vi "Auton Data.vi"(8 "power":dbl[](array[numeric]), 9 "time/distance":dbl[](array[numeric]), 10 "Heading":dbl[](array[numeric]), 11 "primitive ID":i16[](array[numeric])) -> ()   [LabVIEW 2012]
uses:
  <vilib>/Rock Robotics/WPI/DriverStation/DriverStationLCD/WPI_DriverStationLCDLCDLine.ctl
  Begin/Global Variables.vi
panel:
  out "Heading":dbl
  out "Distance/Time":dbl
  out "Power":dbl
  out "ArrayIndex":u16
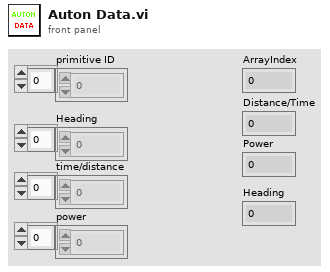
[diagram p1: front panel]
types:
  T1 = typedef "WPI_DriverStationLCDLCDLine.ctl" = enum16{"Main - Line 1", "User - Line 2", "User - Line 3", "User - Line 4", "User - Line 5", "User - Line 6"}
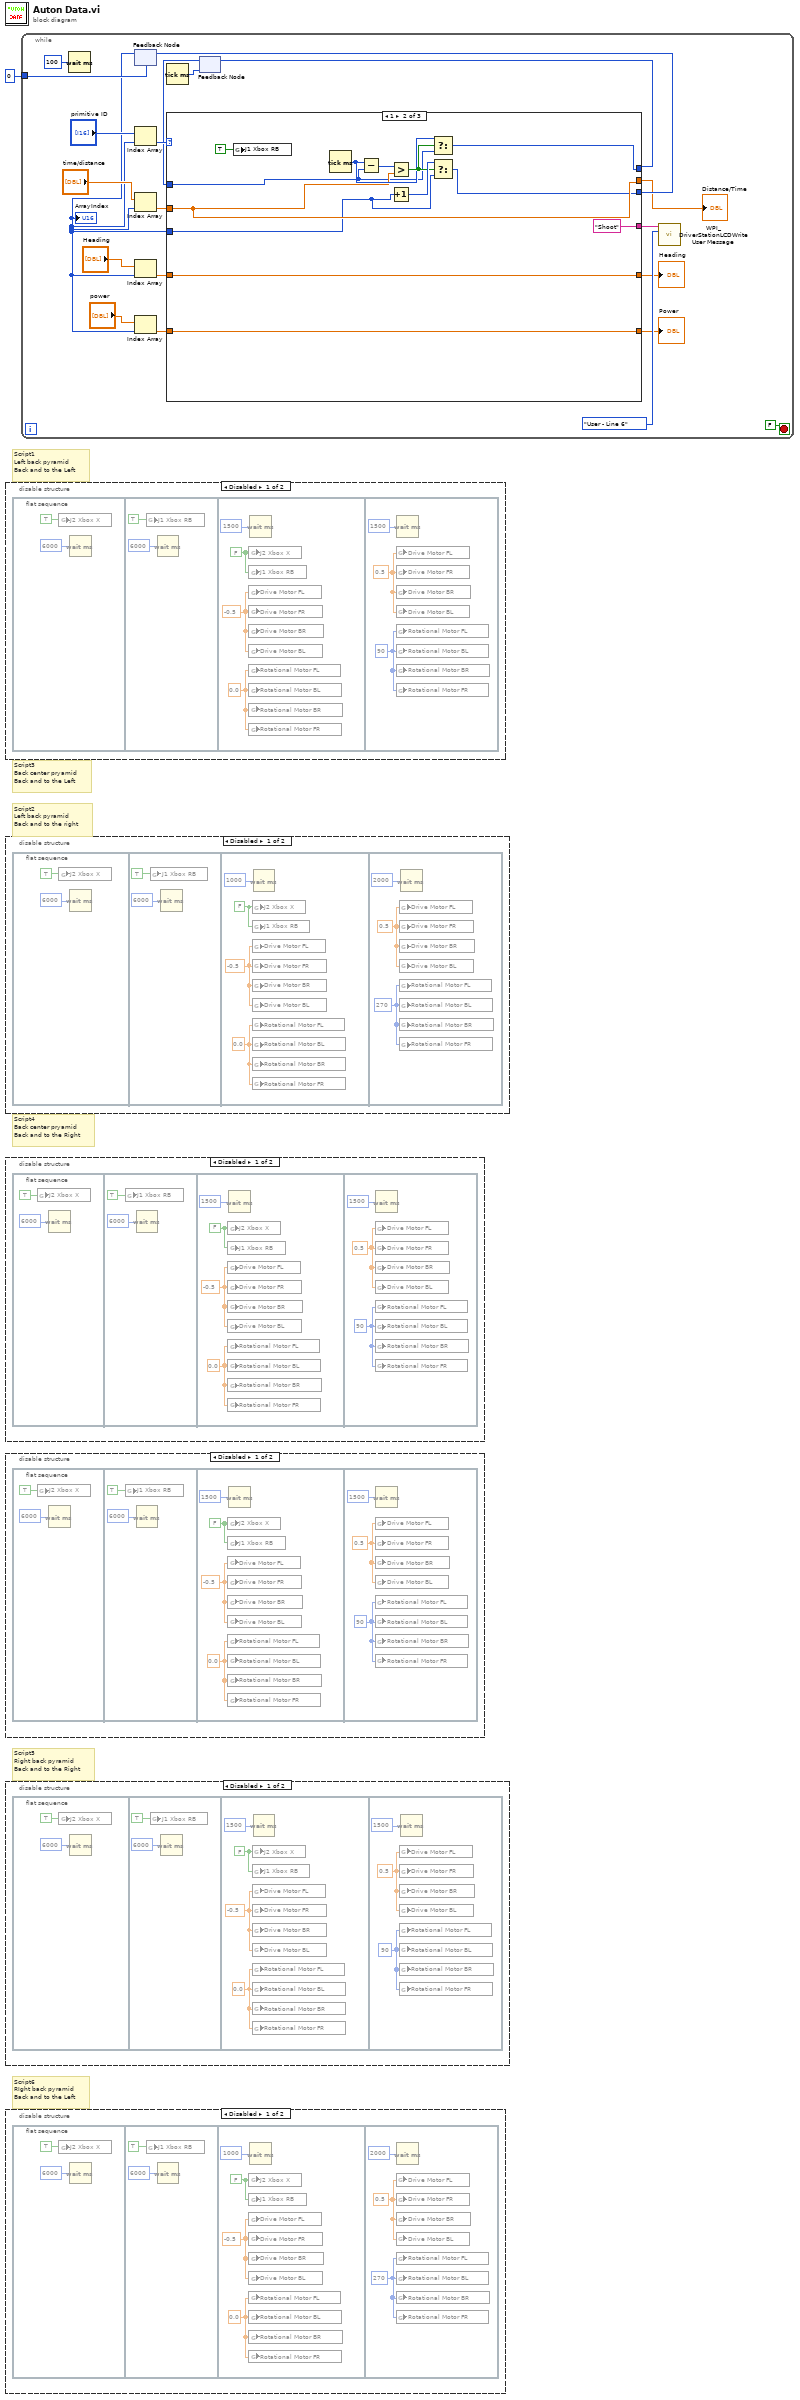
[diagram p0: block diagram]
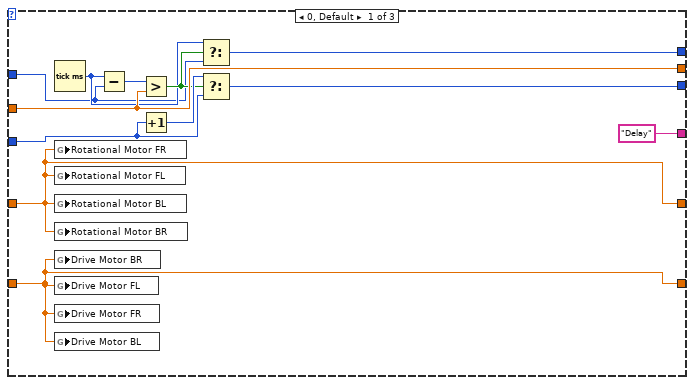
[diagram p2: hidden frame]
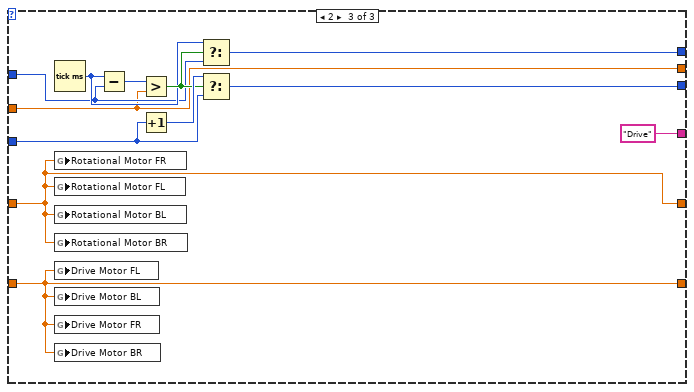
[diagram p3: hidden frame]
diagram:
  # "Script6\nRIght back pyramid\nBack and to the Left"
  # "Script5\nRight back pyramid\nBack and to the Right"
  # "Script4\nBack center pryamid\nBack and to the Right"
  # "Script3\nBack center pryamid\nBack and to the Left"
  # "Script2\nLeft back pyramid\nBack and to the right"
  # "Script1\nLeft back pyramid\nBack and to the Left"
  n1 = disable-structure shown="Disabled" {
    frame Disabled {
      n2 = flat-sequence {
        frame #0 {
          n3 = global write "Global Variables.vi" "J2 Xbox X"(TRUE) -> ()
          n4 = Wait (ms)(milliseconds to wait=u32 6000) -> ()  [unwired: 1 out]
        }
        frame #1 {
          n5 = global write "Global Variables.vi" "J1 Xbox RB"(TRUE ("Shoot trigger")) -> ()
          n6 = Wait (ms)(milliseconds to wait=u32 6000) -> ()  [unwired: 1 out]
        }
        frame #2 {
          w8 = -0.5
          w9 = 0.0
          w6 = FALSE ("Shoot trigger")
          n7 = global write "Global Variables.vi" "J2 Xbox X"(w6) -> ()
          n8 = global write "Global Variables.vi" "J1 Xbox RB"(w6) -> ()
          n9 = global write "Global Variables.vi" "Drive Motor FL"(w8) -> ()
          n10 = global write "Global Variables.vi" "Drive Motor FR"(w8) -> ()
          n11 = global write "Global Variables.vi" "Drive Motor BR"(w8) -> ()
          n12 = global write "Global Variables.vi" "Drive Motor BL"(w8) -> ()
          n13 = global write "Global Variables.vi" "Rotational Motor FL"(w9) -> ()
          n14 = global write "Global Variables.vi" "Rotational Motor BL"(w9) -> ()
          n15 = global write "Global Variables.vi" "Rotational Motor BR"(w9) -> ()
          n16 = global write "Global Variables.vi" "Rotational Motor FR"(w9) -> ()
          n17 = Wait (ms)(milliseconds to wait=u32 1500) -> ()  [unwired: 1 out]
        }
        frame #3 {
          w11 = 0.5
          w10 = 90
          n18 = global write "Global Variables.vi" "Drive Motor FL"(w11) -> ()
          n19 = global write "Global Variables.vi" "Drive Motor FR"(w11) -> ()
          n20 = global write "Global Variables.vi" "Drive Motor BR"(w11) -> ()
          n21 = global write "Global Variables.vi" "Drive Motor BL"(w11) -> ()
          n22 = global write "Global Variables.vi" "Rotational Motor FL"(w10) -> ()
          n23 = global write "Global Variables.vi" "Rotational Motor BL"(w10) -> ()
          n24 = global write "Global Variables.vi" "Rotational Motor BR"(w10) -> ()
          n25 = global write "Global Variables.vi" "Rotational Motor FR"(w10) -> ()
          n26 = Wait (ms)(milliseconds to wait=u32 1500) -> ()  [unwired: 1 out]
        }
      }
    }
    frame Enabled {
    }
  }
  n27 = disable-structure shown="Disabled" {
    frame Disabled {
      n28 = flat-sequence {
        frame #0 {
          n29 = global write "Global Variables.vi" "J2 Xbox X"(TRUE) -> ()
          n30 = Wait (ms)(milliseconds to wait=u32 6000) -> ()  [unwired: 1 out]
        }
        frame #1 {
          n31 = global write "Global Variables.vi" "J1 Xbox RB"(TRUE ("Shoot trigger")) -> ()
          n32 = Wait (ms)(milliseconds to wait=u32 6000) -> ()  [unwired: 1 out]
        }
        frame #2 {
          w19 = -0.5
          w20 = 0.0
          w17 = FALSE ("Shoot trigger")
          n33 = global write "Global Variables.vi" "J2 Xbox X"(w17) -> ()
          n34 = global write "Global Variables.vi" "J1 Xbox RB"(w17) -> ()
          n35 = global write "Global Variables.vi" "Drive Motor FL"(w19) -> ()
          n36 = global write "Global Variables.vi" "Drive Motor FR"(w19) -> ()
          n37 = global write "Global Variables.vi" "Drive Motor BR"(w19) -> ()
          n38 = global write "Global Variables.vi" "Drive Motor BL"(w19) -> ()
          n39 = global write "Global Variables.vi" "Rotational Motor FL"(w20) -> ()
          n40 = global write "Global Variables.vi" "Rotational Motor BL"(w20) -> ()
          n41 = global write "Global Variables.vi" "Rotational Motor BR"(w20) -> ()
          n42 = global write "Global Variables.vi" "Rotational Motor FR"(w20) -> ()
          n43 = Wait (ms)(milliseconds to wait=u32 1000) -> ()  [unwired: 1 out]
        }
        frame #3 {
          w22 = 0.5
          w21 = 270
          n44 = global write "Global Variables.vi" "Drive Motor FL"(w22) -> ()
          n45 = global write "Global Variables.vi" "Drive Motor FR"(w22) -> ()
          n46 = global write "Global Variables.vi" "Drive Motor BR"(w22) -> ()
          n47 = global write "Global Variables.vi" "Drive Motor BL"(w22) -> ()
          n48 = global write "Global Variables.vi" "Rotational Motor FL"(w21) -> ()
          n49 = global write "Global Variables.vi" "Rotational Motor BL"(w21) -> ()
          n50 = global write "Global Variables.vi" "Rotational Motor BR"(w21) -> ()
          n51 = global write "Global Variables.vi" "Rotational Motor FR"(w21) -> ()
          n52 = Wait (ms)(milliseconds to wait=u32 2000) -> ()  [unwired: 1 out]
        }
      }
    }
    frame Enabled {
    }
  }
  n53 = disable-structure shown="Disabled" {
    frame Disabled {
      n54 = flat-sequence {
        frame #0 {
          n55 = global write "Global Variables.vi" "J2 Xbox X"(TRUE) -> ()
          n56 = Wait (ms)(milliseconds to wait=u32 6000) -> ()  [unwired: 1 out]
        }
        frame #1 {
          n57 = global write "Global Variables.vi" "J1 Xbox RB"(TRUE ("Shoot trigger")) -> ()
          n58 = Wait (ms)(milliseconds to wait=u32 6000) -> ()  [unwired: 1 out]
        }
        frame #2 {
          w30 = -0.5
          w31 = 0.0
          w28 = FALSE ("Shoot trigger")
          n59 = global write "Global Variables.vi" "J2 Xbox X"(w28) -> ()
          n60 = global write "Global Variables.vi" "J1 Xbox RB"(w28) -> ()
          n61 = global write "Global Variables.vi" "Drive Motor FL"(w30) -> ()
          n62 = global write "Global Variables.vi" "Drive Motor FR"(w30) -> ()
          n63 = global write "Global Variables.vi" "Drive Motor BR"(w30) -> ()
          n64 = global write "Global Variables.vi" "Drive Motor BL"(w30) -> ()
          n65 = global write "Global Variables.vi" "Rotational Motor FL"(w31) -> ()
          n66 = global write "Global Variables.vi" "Rotational Motor BL"(w31) -> ()
          n67 = global write "Global Variables.vi" "Rotational Motor BR"(w31) -> ()
          n68 = global write "Global Variables.vi" "Rotational Motor FR"(w31) -> ()
          n69 = Wait (ms)(milliseconds to wait=u32 1500) -> ()  [unwired: 1 out]
        }
        frame #3 {
          w33 = 0.5
          w32 = 90
          n70 = global write "Global Variables.vi" "Drive Motor FL"(w33) -> ()
          n71 = global write "Global Variables.vi" "Drive Motor FR"(w33) -> ()
          n72 = global write "Global Variables.vi" "Drive Motor BR"(w33) -> ()
          n73 = global write "Global Variables.vi" "Drive Motor BL"(w33) -> ()
          n74 = global write "Global Variables.vi" "Rotational Motor FL"(w32) -> ()
          n75 = global write "Global Variables.vi" "Rotational Motor BL"(w32) -> ()
          n76 = global write "Global Variables.vi" "Rotational Motor BR"(w32) -> ()
          n77 = global write "Global Variables.vi" "Rotational Motor FR"(w32) -> ()
          n78 = Wait (ms)(milliseconds to wait=u32 1500) -> ()  [unwired: 1 out]
        }
      }
    }
    frame Enabled {
    }
  }
  n79 = disable-structure shown="Disabled" {
    frame Disabled {
      n80 = flat-sequence {
        frame #0 {
          n81 = global write "Global Variables.vi" "J2 Xbox X"(TRUE) -> ()
          n82 = Wait (ms)(milliseconds to wait=u32 6000) -> ()  [unwired: 1 out]
        }
        frame #1 {
          n83 = global write "Global Variables.vi" "J1 Xbox RB"(TRUE ("Shoot trigger")) -> ()
          n84 = Wait (ms)(milliseconds to wait=u32 6000) -> ()  [unwired: 1 out]
        }
        frame #2 {
          w41 = -0.5
          w42 = 0.0
          w39 = FALSE ("Shoot trigger")
          n85 = global write "Global Variables.vi" "J2 Xbox X"(w39) -> ()
          n86 = global write "Global Variables.vi" "J1 Xbox RB"(w39) -> ()
          n87 = global write "Global Variables.vi" "Drive Motor FL"(w41) -> ()
          n88 = global write "Global Variables.vi" "Drive Motor FR"(w41) -> ()
          n89 = global write "Global Variables.vi" "Drive Motor BR"(w41) -> ()
          n90 = global write "Global Variables.vi" "Drive Motor BL"(w41) -> ()
          n91 = global write "Global Variables.vi" "Rotational Motor FL"(w42) -> ()
          n92 = global write "Global Variables.vi" "Rotational Motor BL"(w42) -> ()
          n93 = global write "Global Variables.vi" "Rotational Motor BR"(w42) -> ()
          n94 = global write "Global Variables.vi" "Rotational Motor FR"(w42) -> ()
          n95 = Wait (ms)(milliseconds to wait=u32 1500) -> ()  [unwired: 1 out]
        }
        frame #3 {
          w44 = 0.5
          w43 = 90
          n96 = global write "Global Variables.vi" "Drive Motor FL"(w44) -> ()
          n97 = global write "Global Variables.vi" "Drive Motor FR"(w44) -> ()
          n98 = global write "Global Variables.vi" "Drive Motor BR"(w44) -> ()
          n99 = global write "Global Variables.vi" "Drive Motor BL"(w44) -> ()
          n100 = global write "Global Variables.vi" "Rotational Motor FL"(w43) -> ()
          n101 = global write "Global Variables.vi" "Rotational Motor BL"(w43) -> ()
          n102 = global write "Global Variables.vi" "Rotational Motor BR"(w43) -> ()
          n103 = global write "Global Variables.vi" "Rotational Motor FR"(w43) -> ()
          n104 = Wait (ms)(milliseconds to wait=u32 1500) -> ()  [unwired: 1 out]
        }
      }
    }
    frame Enabled {
    }
  }
  n105 = disable-structure shown="Disabled" {
    frame Disabled {
      n106 = flat-sequence {
        frame #0 {
          n107 = global write "Global Variables.vi" "J2 Xbox X"(TRUE) -> ()
          n108 = Wait (ms)(milliseconds to wait=u32 6000) -> ()  [unwired: 1 out]
        }
        frame #1 {
          n109 = global write "Global Variables.vi" "J1 Xbox RB"(TRUE ("Shoot trigger")) -> ()
          n110 = Wait (ms)(milliseconds to wait=u32 6000) -> ()  [unwired: 1 out]
        }
        frame #2 {
          w52 = -0.5
          w53 = 0.0
          w50 = FALSE ("Shoot trigger")
          n111 = global write "Global Variables.vi" "J2 Xbox X"(w50) -> ()
          n112 = global write "Global Variables.vi" "J1 Xbox RB"(w50) -> ()
          n113 = global write "Global Variables.vi" "Drive Motor FL"(w52) -> ()
          n114 = global write "Global Variables.vi" "Drive Motor FR"(w52) -> ()
          n115 = global write "Global Variables.vi" "Drive Motor BR"(w52) -> ()
          n116 = global write "Global Variables.vi" "Drive Motor BL"(w52) -> ()
          n117 = global write "Global Variables.vi" "Rotational Motor FL"(w53) -> ()
          n118 = global write "Global Variables.vi" "Rotational Motor BL"(w53) -> ()
          n119 = global write "Global Variables.vi" "Rotational Motor BR"(w53) -> ()
          n120 = global write "Global Variables.vi" "Rotational Motor FR"(w53) -> ()
          n121 = Wait (ms)(milliseconds to wait=u32 1500) -> ()  [unwired: 1 out]
        }
        frame #3 {
          w55 = 0.5
          w54 = 90
          n122 = global write "Global Variables.vi" "Drive Motor FL"(w55) -> ()
          n123 = global write "Global Variables.vi" "Drive Motor FR"(w55) -> ()
          n124 = global write "Global Variables.vi" "Drive Motor BR"(w55) -> ()
          n125 = global write "Global Variables.vi" "Drive Motor BL"(w55) -> ()
          n126 = global write "Global Variables.vi" "Rotational Motor FL"(w54) -> ()
          n127 = global write "Global Variables.vi" "Rotational Motor BL"(w54) -> ()
          n128 = global write "Global Variables.vi" "Rotational Motor BR"(w54) -> ()
          n129 = global write "Global Variables.vi" "Rotational Motor FR"(w54) -> ()
          n130 = Wait (ms)(milliseconds to wait=u32 1500) -> ()  [unwired: 1 out]
        }
      }
    }
    frame Enabled {
    }
  }
  n131 = disable-structure shown="Disabled" {
    frame Disabled {
      n132 = flat-sequence {
        frame #0 {
          n133 = global write "Global Variables.vi" "J2 Xbox X"(TRUE) -> ()
          n134 = Wait (ms)(milliseconds to wait=u32 6000) -> ()  [unwired: 1 out]
        }
        frame #1 {
          n135 = global write "Global Variables.vi" "J1 Xbox RB"(TRUE ("Shoot trigger")) -> ()
          n136 = Wait (ms)(milliseconds to wait=u32 6000) -> ()  [unwired: 1 out]
        }
        frame #2 {
          w63 = -0.5
          w64 = 0.0
          w61 = FALSE ("Shoot trigger")
          n137 = global write "Global Variables.vi" "J2 Xbox X"(w61) -> ()
          n138 = global write "Global Variables.vi" "J1 Xbox RB"(w61) -> ()
          n139 = global write "Global Variables.vi" "Drive Motor FL"(w63) -> ()
          n140 = global write "Global Variables.vi" "Drive Motor FR"(w63) -> ()
          n141 = global write "Global Variables.vi" "Drive Motor BR"(w63) -> ()
          n142 = global write "Global Variables.vi" "Drive Motor BL"(w63) -> ()
          n143 = global write "Global Variables.vi" "Rotational Motor FL"(w64) -> ()
          n144 = global write "Global Variables.vi" "Rotational Motor BL"(w64) -> ()
          n145 = global write "Global Variables.vi" "Rotational Motor BR"(w64) -> ()
          n146 = global write "Global Variables.vi" "Rotational Motor FR"(w64) -> ()
          n147 = Wait (ms)(milliseconds to wait=u32 1000) -> ()  [unwired: 1 out]
        }
        frame #3 {
          w66 = 0.5
          w65 = 270
          n148 = global write "Global Variables.vi" "Drive Motor FL"(w66) -> ()
          n149 = global write "Global Variables.vi" "Drive Motor FR"(w66) -> ()
          n150 = global write "Global Variables.vi" "Drive Motor BR"(w66) -> ()
          n151 = global write "Global Variables.vi" "Drive Motor BL"(w66) -> ()
          n152 = global write "Global Variables.vi" "Rotational Motor FL"(w65) -> ()
          n153 = global write "Global Variables.vi" "Rotational Motor BL"(w65) -> ()
          n154 = global write "Global Variables.vi" "Rotational Motor BR"(w65) -> ()
          n155 = global write "Global Variables.vi" "Rotational Motor FR"(w65) -> ()
          n156 = Wait (ms)(milliseconds to wait=u32 2000) -> ()  [unwired: 1 out]
        }
      }
    }
    frame Enabled {
    }
  }
  n157 = while {
    tunnel: 0 -> [w81]
    stop <- FALSE stop-if-true
    n158 = Wait (ms)(milliseconds to wait=u32 100) -> ()  [unwired: 1 out]
    n159 = feedback #1(w81) -> (w71:i32)
    "ArrayIndex" <- w71
    n160 = Index Array(array="primitive ID", index=w71) -> (element=w72:i16)
    n161 = Index Array(array="time/distance", index=w71) -> (element=w75:dbl)
    n162 = Index Array(array="Heading", index=w71) -> (element=w73:dbl)
    n163 = Index Array(array="power", index=w71) -> (element=w77:dbl)
    n164 = Tick Count (ms)() -> (millisecond timer value=w70:u32)
    n165 = feedback #2(w70) -> (w69:u32)
    n166 = case shown="1" w72 {
      tunnel: ["Delay" ("line text") "Shoot" ("line text") "Drive" ("line text")] -> w80
      tunnel: [w97 w101 w114] -> w79
      tunnel: [w90 w112 w123] -> w78
      tunnel: w77 -> [w90 w112 w123]
      tunnel: [w98 w105 w116] -> w76
      tunnel: w75 -> [w98 w105 w116]
      tunnel: [w89 w111 w124] -> w74
      tunnel: w73 -> [w89 w111 w124]
      tunnel: w71 -> [w95 w104 w115]
      tunnel: w69 -> [w92 w103 w118]
      tunnel: [w91 w102 w117] -> w68
      frame 0, Default {
        n167 = Tick Count (ms)() -> (millisecond timer value=w93:u32)
        n168 = global write "Global Variables.vi" "Rotational Motor FR"(w89) -> ()
        n169 = global write "Global Variables.vi" "Rotational Motor FL"(w89) -> ()
        n170 = global write "Global Variables.vi" "Rotational Motor BL"(w89) -> ()
        n171 = global write "Global Variables.vi" "Rotational Motor BR"(w89) -> ()
        n172 = global write "Global Variables.vi" "Drive Motor BR"(w90) -> ()
        n173 = global write "Global Variables.vi" "Drive Motor FL"(w90) -> ()
        n174 = global write "Global Variables.vi" "Drive Motor FR"(w90) -> ()
        n175 = global write "Global Variables.vi" "Drive Motor BL"(w90) -> ()
        n176 = Subtract(x=w93, y=w92) -> (x-y=w99:u32)
        n177 = Greater?(x=w99, y=w98) -> (0:w94:bool)
        n178 = Increment(x=w95) -> (x+1=w96:i32)
        n179 = Select(t=w93, s=w94, f=w92) -> (s? t:f=w91:u32)
        n180 = Select(t=w96, s=w94, f=w95) -> (s? t:f=w97:i32)
      }
      frame 1 {
        n181 = global write "Global Variables.vi" "J1 Xbox RB"(TRUE ("Shoot trigger")) -> ()
        n182 = Tick Count (ms)() -> (millisecond timer value=w106:u32)
        n183 = Subtract(x=w106, y=w103) -> (x-y=w109:u32)
        n184 = Greater?(x=w109, y=w105) -> (0:w107:bool)
        n185 = Increment(x=w104) -> (x+1=w108:i32)
        n186 = Select(t=w106, s=w107, f=w103) -> (s? t:f=w102:u32)
        n187 = Select(t=w108, s=w107, f=w104) -> (s? t:f=w101:i32)
      }
      frame 2 {
        n188 = Tick Count (ms)() -> (millisecond timer value=w119:u32)
        n189 = global write "Global Variables.vi" "Rotational Motor FR"(w124) -> ()
        n190 = global write "Global Variables.vi" "Rotational Motor FL"(w124) -> ()
        n191 = global write "Global Variables.vi" "Rotational Motor BL"(w124) -> ()
        n192 = global write "Global Variables.vi" "Rotational Motor BR"(w124) -> ()
        n193 = global write "Global Variables.vi" "Drive Motor FL"(w123) -> ()
        n194 = global write "Global Variables.vi" "Drive Motor BL"(w123) -> ()
        n195 = global write "Global Variables.vi" "Drive Motor FR"(w123) -> ()
        n196 = global write "Global Variables.vi" "Drive Motor BR"(w123) -> ()
        n197 = Subtract(x=w119, y=w118) -> (x-y=w122:u32)
        n198 = Greater?(x=w122, y=w116) -> (0:w120:bool)
        n199 = Increment(x=w115) -> (x+1=w121:i32)
        n200 = Select(t=w119, s=w120, f=w118) -> (s? t:f=w117:u32)
        n201 = Select(t=w121, s=w120, f=w115) -> (s? t:f=w114:i32)
      }
    }
    "Heading" <- w74
    "Distance/Time" <- w76
    "Power" <- w78
    n202 = feedback-in #1(w79) -> ()
    n203 = feedback-in #2(w68) -> ()
    n204 = call <vilib>:"WPI_DriverStationLCDWrite User Message.vi"("line text"=w80, "line"=WPI_DriverStationLCDLCDLine."User - Line 6") -> ()  [unwired: 13 in, 1 out]
  }
